vi "BotSpeak_AddCmd.vi"(2 "String":string, 3 "URAPI Script":T1) -> (1 "URAPI Script out":T1)   [LabVIEW 2014]
uses:
  <userlib>/botspeak/VIs/Direct/URAPI_Control.ctl
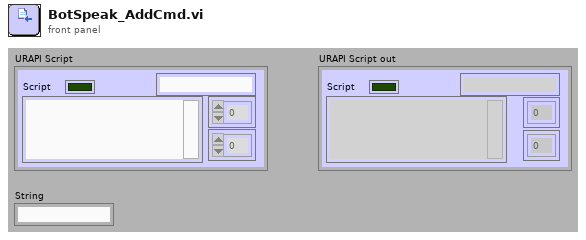
[diagram p1: front panel]
types:
  T1 = typedef "URAPI_Control.ctl" = cluster{"Script":string, "Whiles":u8[], "Ifs":u8[], "Supress Err":bool, "Errors":string}
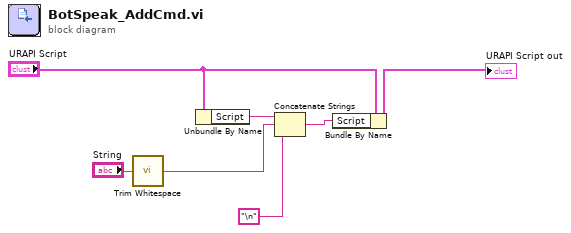
[diagram p0: block diagram]
diagram:
  n1 = call <vilib>:"Trim Whitespace.vi"("string"="String") -> ("trimmed string"=w2:string)  [unwired: 1 in]
  n2 = Unbundle By Name("URAPI Script") -> ("Script"=w5:string)
  n3 = Concatenate Strings(w5, w2, "\n" ("String")) -> (w6:string)
  n4 = Bundle By Name(cluster="URAPI Script", "Script"=w6) -> (→"URAPI Script out":T1)
